vi "显示曲线.vi"(2 "力觉参数":T1={"选择"=enum."Fx", "系数"=1.0, "上限"=2.55, "下限"=2.05, "Ymax"=5.0, "Ymin"=-5.0, "点数"=1000.0, "起点"=0.0, "终点"=0.0} {"终点" format="%.2f"; "起点" format="%.2f"; "下限" format="%.2f"; "上限" format="%.2f"; "系数" format="%.3f"}, 3 "力数组":sgl[](array[numeric]) format="%.2f") -> (1 "力值":sgl format="%.3f")   [LabVIEW 2018]
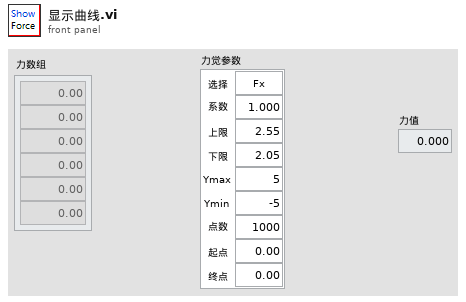
[diagram p1: front panel]
types:
  T1 = cluster{"选择":enum16{"Fx", "Fy", "Fz", "Mx", "My", "Mz"}, "系数":sgl, "上限":sgl, "下限":sgl, "Ymax":dbl, "Ymin":dbl, "点数":dbl, "起点":dbl, "终点":dbl}
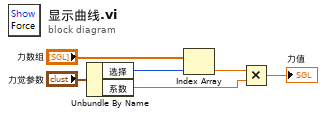
[diagram p0: block diagram]
diagram:
  n1 = Unbundle By Name("力觉参数") -> ("选择"=w6:enum16{"Fx", "Fy", "Fz", "Mx", "My", "Mz"}, "系数"=w4:sgl)
  n2 = Index Array(array="力数组", index=w6) -> (element=w5:sgl)
  n3 = Multiply(x=w5, y=w4) -> (x*y=→"力值":sgl)
